vi "Extract Single Tone Information 1 Chan (CDB).vi"(6 "advanced search":T1={"approx freq. (optional)"=nan, "search (+/- % of Fsampl.)"=5.0} {"search (+/- % of Fsampl.)" format="%0.2p"; "approx freq. (optional)" format="%0.2p"}, 8 "error in (no error)":errorcluster, 10 "export mode":T2(ring), 11 "time signal in":waveform(cdb)) -> (0 "error out":errorcluster, 1 "detected phase (deg)":dbl format="%.2p", 2 "detected amplitude":dbl format="%.2p", 3 "detected frequency":dbl format="%.2p", 4 "measurement info":T3={"uncertainty"=0.0, "Warning"=FALSE, "comments"="reserved for future use"} {"uncertainty" format="%0.2p"}, 5 "exported signals":T4 {"exported spectrum (dB)"."dB Spectrum (Hann)" format="%.2p"; "exported spectrum (dB)"."df" format="%.2p"; "exported spectrum (dB)"."f0" format="%.2p"})   [LabVIEW 2020, in "NI_MAPro.lvlib"]
doc: "Takes a signal in, finds the single tone with the highest amplitude or searches a specified frequency range, and returns the single tone frequency, amplitude, and phase. The input signal can be real or complex and single-channel or multichannel. Wire data to the <B>time signal in</B> input to determine the polymorphic instance to use or manually select the instance."
uses:
  NI_MAPro.lvlib
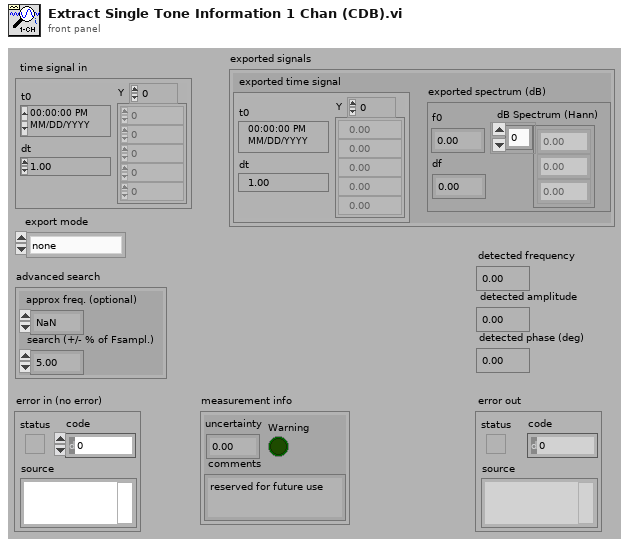
[diagram p1: front panel]
types:
  T1 = cluster{"approx freq. (optional)":dbl, "search (+/- % of Fsampl.)":dbl}
  T2 = enum32{"none", "input signal", "detected signal", "residual signal"}
  T3 = cluster{"uncertainty":dbl, "Warning":bool, "comments":string}
  T4 = cluster{"exported time signal":waveform(cdb), "exported spectrum (dB)":cluster{"f0":dbl, "df":dbl, "dB Spectrum (Hann)":dbl[]}}
  T5 = typedef "NI_MAPro.lvlib/ma_sml_Spectral Info.ctl" = cluster{"spectrum type":enum16{"FFT Spectrum [complex]", "Amplitude [Magnitude]", "Power [Magnitude^2]", "Cross Spectrum [complex]", "Frequency Response [Complex]"}, "linear/dB":enum16{"linear", "dB"}, "window":u16, "window size":i32, "FFT size":i32}
  T6 = typedef "NI_MAPro.lvlib/ma_sml_Spectrum Cluster (complex).ctl" = cluster{"f0":dbl, "df":dbl, "spectrum":cdb[]}
  T7 = cluster{"frequency":dbl, "amplitude":dbl, "phase [degree]":dbl}
  T8 = cluster{"time signal in":waveform(cdb), cluster{dbl, dbl, "Y":dbl[]}}
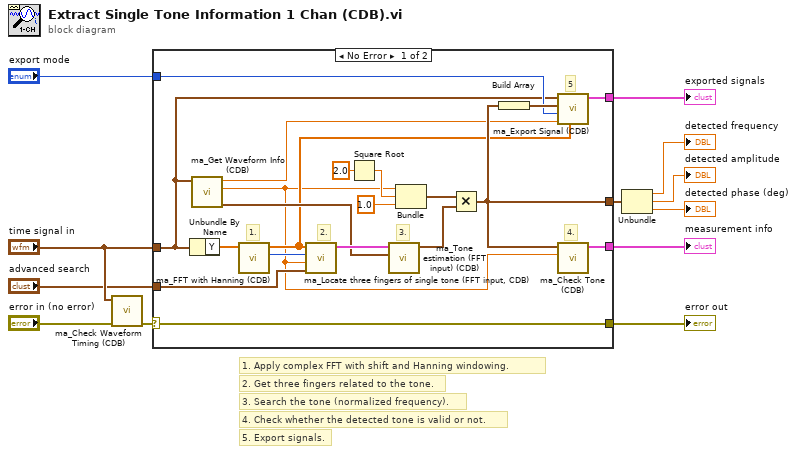
[diagram p0: block diagram]
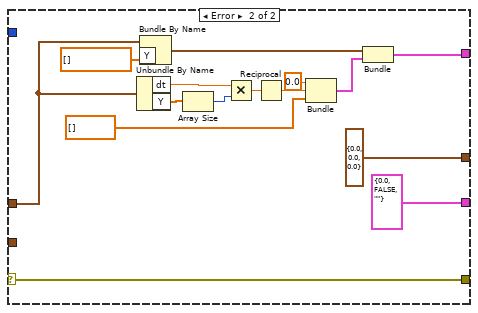
[diagram p2: hidden frame]
diagram:
  # "5. Export signals."
  # "4. Check whether the detected tone is valid or not."
  # "3. Search the tone (normalized frequency)."
  # "2. Get three fingers related to the tone."
  # "1. Apply complex FFT with shift and Hanning windowing."
  n1 = call "ma_Check Waveform Timing (CDB).vi"("error in (no error)"="error in (no error)", "signal in"="time signal in") -> ("error out"=w9:errorcluster)  [unwired: 1 in, 8 out]
  n2 = case shown="No Error" w9 {
    selector: w9 -> [w31 w47]
    tunnel: "time signal in" -> [w17 w34]
    tunnel: [w31 w47] -> w12
    tunnel: [w22 cluster{dbl, dbl, dbl} {0.0, 0.0, 0.0}] -> w8
    tunnel: "export mode" -> [w24 _]
    tunnel: [w23 w33] -> w3
    tunnel: [w21 cluster{dbl, bool, string} {0.0, FALSE, ""}] -> w2
    tunnel: "advanced search" -> [w19 _]
    frame No Error {
      # "5"
      # "4."
      # "3."
      # "2."
      # "1."
      n3 = Unbundle By Name(w17) -> ("Y"=w32:cdb[])
      n4 = call "ma_Get Waveform Info (CDB).vi"("time signal in"=w17) -> ("spectral info"=w15:T5, "fs"=w13:dbl, "f0"=w16:dbl)  [unwired: 8 out]
      n5 = call "ma_FFT with Hanning (CDB).vi"("time signal data"=w32) -> ("FFT size"=w20:i32, "complex Hann spectrum"=w14:cdb[])  [unwired: 9 out]
      n6 = call "ma_Locate three fingers of single tone (FFT input, CDB).vi"("advanced search"=w19, "fs"=w13, "FFT size"=w20, "Complex  Hann spectrum"=w14) -> ("three fingers"=w18:T6)  [unwired: 7 out]
      n7 = Square Root(x=2.0) -> (sqrt(x)=w26:dbl)
      n8 = call "ma_Tone estimation (FFT input) (CDB).vi"("spectral info"=w15, "three fingers"=w18) -> ("single tone info."=w28:T7)  [unwired: 9 out]
      n9 = Bundle("fs"=w13, w26, "x*y"=1.0) -> (w29:cluster{"fs":dbl, dbl, "x*y":dbl})  [unwired: 1 out]
      n10 = Multiply(x=w29, y=w28) -> (x*y=w22:cluster{dbl, dbl, dbl})
      n11 = Build Array(w22) -> (w25:cluster{dbl, dbl, dbl}[])
      n12 = call "ma_Export Signal (CDB).vi"("complex Hann spectrum"=w14, "f0"=w16, "export signals"=w24, "multiple tone information"=w25, "time signal in"=w17) -> ("exported signals"=w23:T4)  [unwired: 1 in, 5 out]
      n13 = call "ma_Check Tone (CDB).vi"("fs"=w13, "tone info"=w22) -> ("measurement info"=w21:T3)  [unwired: 9 out]
    }
    frame Error {
      n14 = Unbundle By Name(w34) -> ("dt"=w37:dbl, "Y"=w39:cdb[])
      n15 = Bundle By Name(cluster=w34, "Y"=cdb[] []) -> (w43:waveform(cdb))
      n16 = Array Size(array=w39) -> (size(s)=w38:i32)
      n17 = Multiply(x=w37, y=w38) -> (x*y=w36:dbl)
      n18 = Reciprocal(x=w36) -> (1/x=w35:dbl)
      n19 = Bundle(0.0, w35, "Y"=dbl[] []) -> (w42:cluster{dbl, dbl, "Y":dbl[]})  [unwired: 1 out]
      n20 = Bundle("time signal in"=w43, w42) -> (w33:T8)  [unwired: 1 out]
    }
  }
  "error out" <- w12
  "exported signals" <- w3
  "measurement info" <- w2
  n21 = Unbundle(w8) -> (→"detected frequency":dbl, →"detected amplitude":dbl, →"detected phase (deg)":dbl)
